vi "CRYProject Editor TS Load Open Sub.vi"(0 "Seq File Name":string, 1 "Sequence path":path) -> (7 "TS Array":T1 {"Steps"."Repeat State Array"."Start" format="%#_5g"; "Steps"."Y dB ref" format="%.1f"; "Steps"."Y data" items=["dB", "Lin"]; "Steps"."Start" format="%#_5g"}, 9 "status":bool)   [LabVIEW 2013]
uses:
  CRYSystem/Typedef Control/CRYTS.ctl
  CRYSystem/Typedef Control/CRYStep.ctl
  CRYSystem/Calibration/SubVI/CRYCal Global.vi
  CRYSystem/Misc/SubVI/CRYMisc vis settings global.vi
  CRYMainGlobal.vi
panel:
  # "Sequence Loading..."
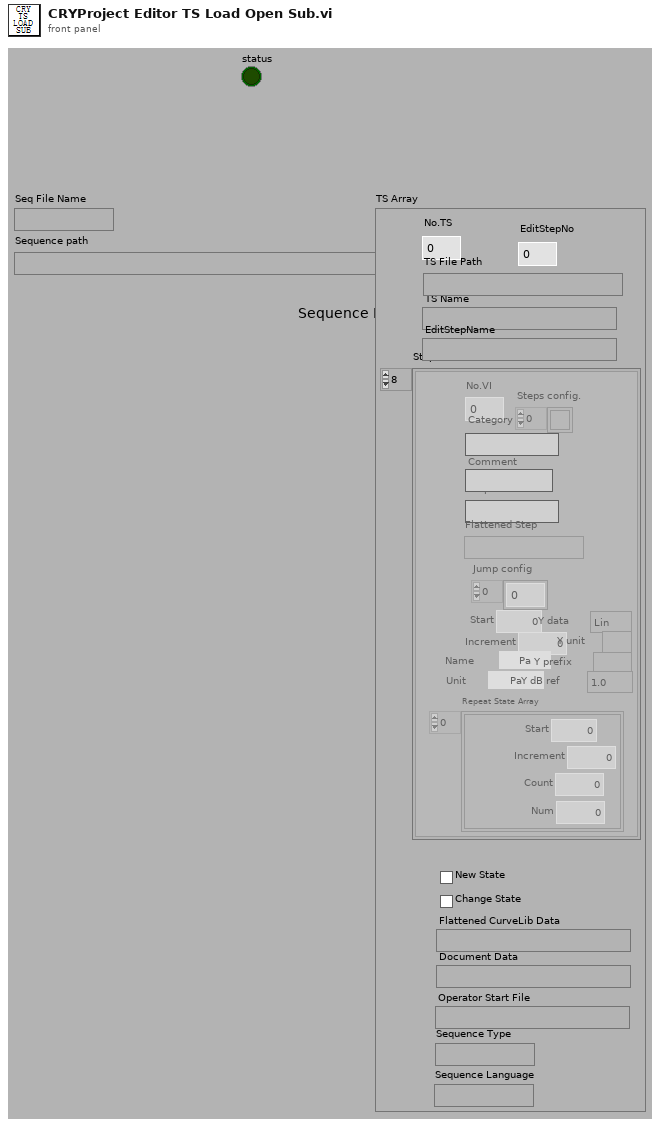
[diagram p1: front panel]
types:
  T1 = typedef "CRYTS.ctl" = cluster{"No.TS":u16, "TS File Path":path, "TS Name":string, "EditStepName":string, "Steps":T2[], "New State":bool, "Change State":bool, "Flattened CurveLib Data":string, "Document Data":string, "EditStepNo":u16, "Operator Start File":string, "Sequence Type":string, "Sequence Language":string}
  T2 = typedef "CRYStep.ctl" = cluster{"No.VI":i32, "Category":string, "StepName":string, "Seq setup flattened":string, "Comment":string, "Steps config.":bool[], "Jump config":i32[], "Start":dbl, "Increment":dbl, "Name":string, "Unit":string, "Y data":u16, "Y prefix":string, "Y dB ref":dbl, "Y unit":string, "Repeat State Array":cluster{"Start":dbl, "Increment":dbl, "Count":i32, "Num":i32}[]}
  T3 = typedef "CRYSequence Cluster.ctl" = cluster{"EditStepName":string, "Trimmed string array":string, "Flattened CurveData":string, "Document Data":string, "EditStepNo":u16, "Operator Start File":path, "Sequence Type":string, "Sequence Language":string, "Sequence Work State":string}
  T4 = cluster{"Data type":string, "Version":u16, "Dimensions":u8}
  T5 = enum16{"OK", "Yes", "YesNo", "YesNoCancel", "ReplaceAppend"}
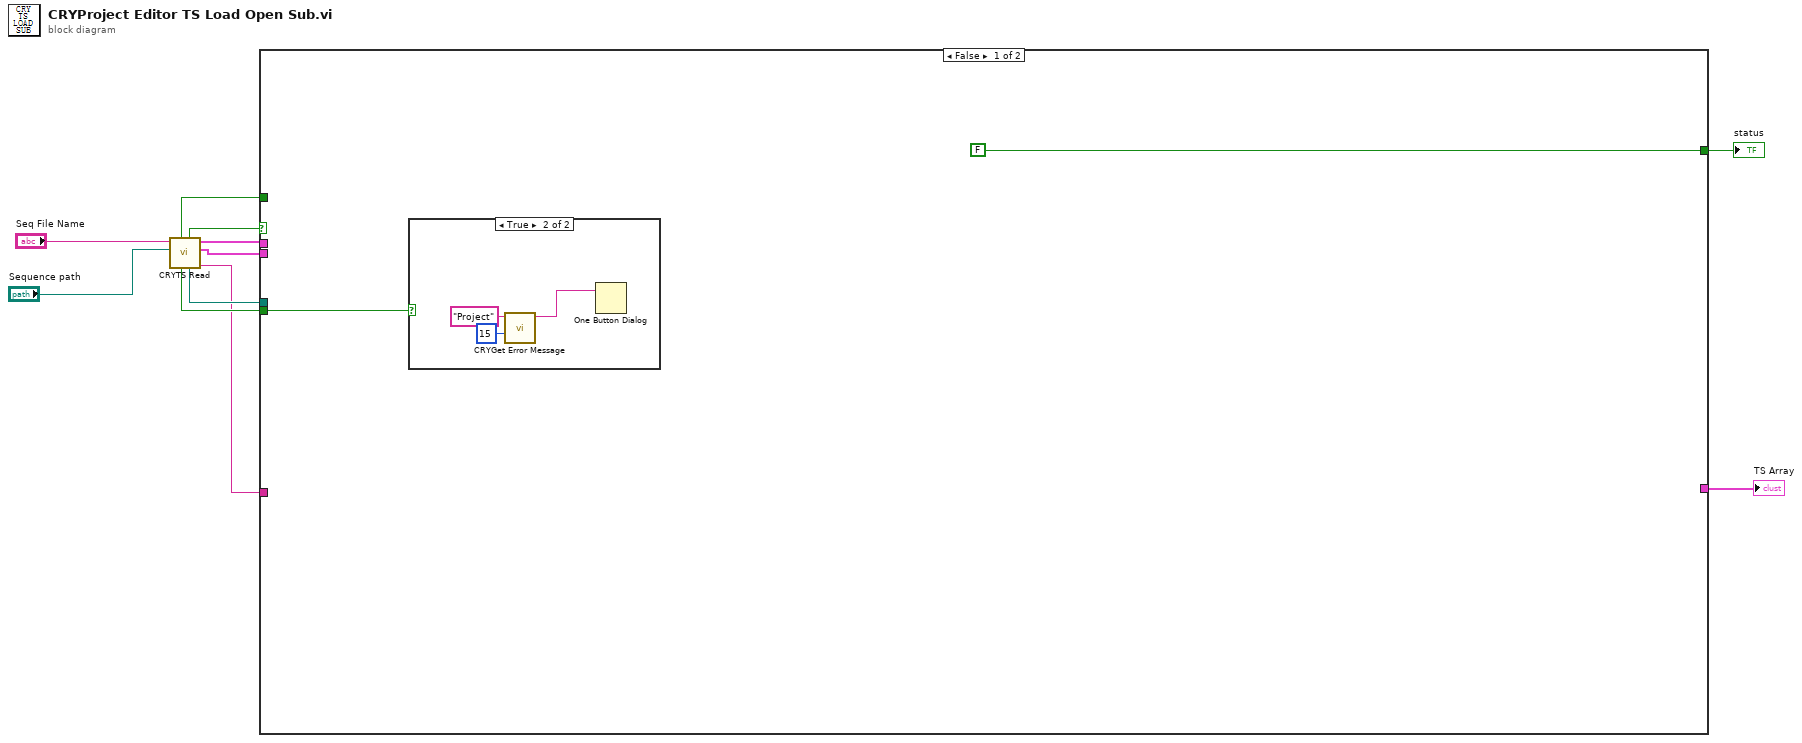
[diagram p0: block diagram]
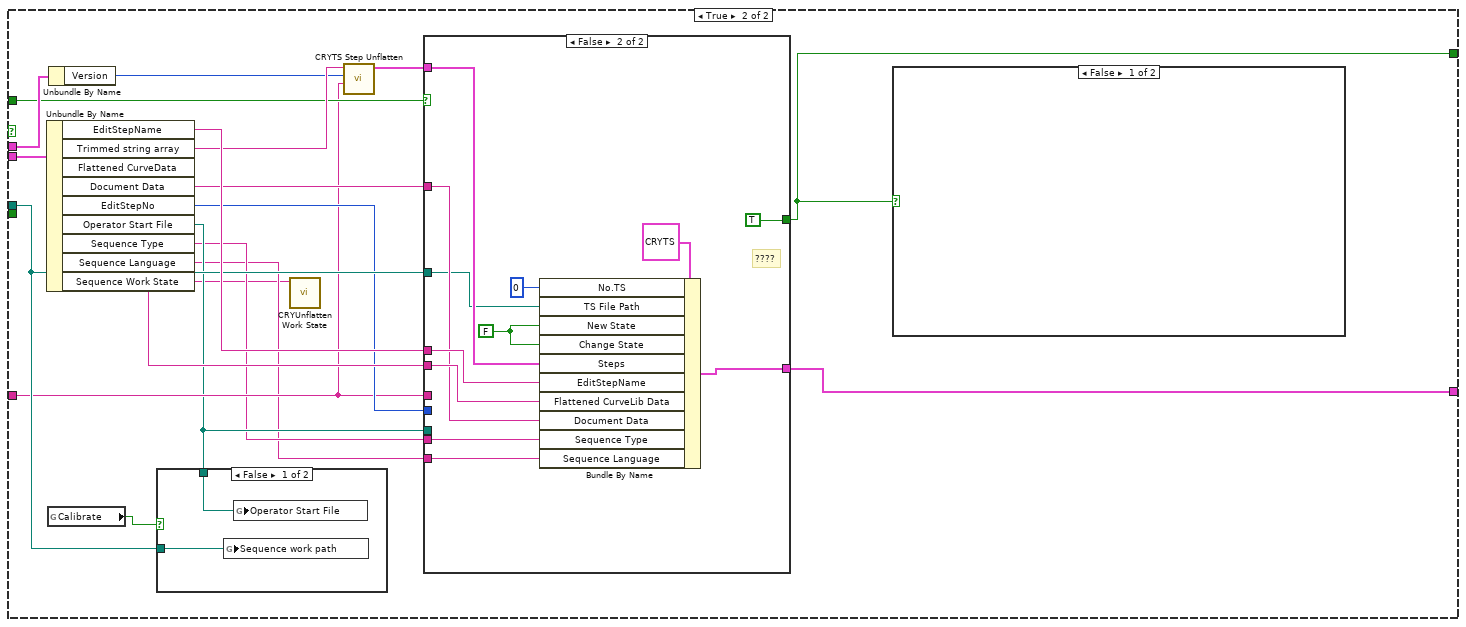
[diagram p3: hidden frame]
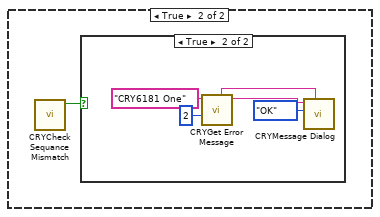
[diagram p5: hidden frame]
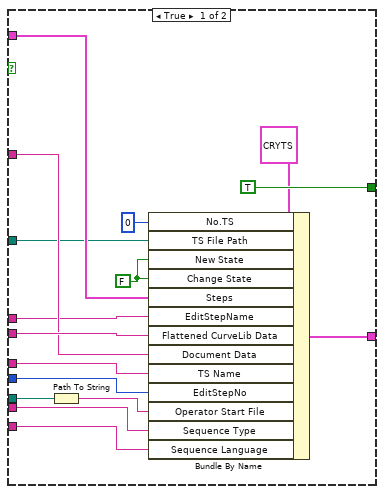
[diagram p7: hidden frame]
diagram:
  n1 = call "CRYTS Read.vi"("Sequence folder path"="Sequence path", "File Name"="Seq File Name") -> ("Sequence Name"=w4:string, "sequence list"=w6:T3, "Header info"=w8:T4, "Selected Seq Path"=w10:path, "status"=w5:bool, "Is RecentFile?"=w9:bool, "Is Replace?"=w7:bool)  [unwired: 3 out]
  n2 = case shown="False" w5 {
    tunnel: w6 -> [_ w35]
    tunnel: [FALSE ("status") w32] -> w11
    tunnel: w10 -> [_ w26]
    tunnel: w9 -> [w12 _]
    tunnel: w8 -> [_ w30]
    tunnel: w7 -> [_ w28]
    tunnel: w4 -> [_ w24]
    tunnel: [_ w17] -> w1
    frame False {
      n3 = case shown="True" w12 {
        frame False {
        }
        frame True {
          n4 = call "CRYGet Error Message.vi"("Error No"=15, "Kind"="Project") -> ("Message"=w14:string)  [unwired: 4 in, 5 out]
          n5 = One Button Dialog(message=w14) -> ()  [unwired: 2 out]
        }
      }
    }
    frame True {
      n6 = Unbundle By Name(w35) -> ("EditStepName"=w34:string, "Trimmed string array"=w31:string, "Flattened CurveData"=w33:string, "Document Data"=w27:string, "EditStepNo"=w25:u16, "Operator Start File"=w23:path, "Sequence Type"=w22:string, "Sequence Language"=w20:string, "Sequence Work State"=w19:string)
      n7 = global read "CRYCal Global.vi" "Calibrate"() -> (w18:bool)
      n8 = Unbundle By Name(w30) -> ("Version"=w29:u16)
      n9 = case shown="False" w18 {
        tunnel: w26 -> [w37 _]
        tunnel: w23 -> [w36 _]
        frame False {
          n10 = global write "CRYMainGlobal.vi" "Sequence work path"(w37) -> ()
          n11 = global write "CRYMisc vis settings global.vi" "Operator Start File"(w36) -> ()
        }
        frame True {
        }
      }
      n12 = call "CRYUnflatten Work State.vi"("Unflatten work state #"=w19) -> ()  [unwired: 9 in, 2 out]
      n13 = call "CRYTS Step Unflatten.vi"("Sequence Name"=w24, "Version"=w29, "Flattened Steps"=w31) -> ("Unflattened Steps"=w21:T2[])  [unwired: 8 out]
      n14 = case shown="False" w28 {
        tunnel: w21 -> [w59 w70]
        tunnel: [w51 w62] -> w17
        tunnel: w34 -> [w48 w68]
        tunnel: w33 -> [w58 w67]
        tunnel: [TRUE TRUE] -> w32
        tunnel: w27 -> [w53 w64]
        tunnel: w26 -> [w52 w63]
        tunnel: w24 -> [w50 _]
        tunnel: w25 -> [w49 _]
        tunnel: w23 -> [w47 _]
        tunnel: w22 -> [w45 w61]
        tunnel: w20 -> [w44 w60]
        frame True {
          w56 = FALSE ("New Sequence Flag")
          n15 = Path To String(path=w47) -> (string=w46:string)
          n16 = Bundle By Name(cluster=T1 {"No.TS"=0, "TS File Path"=path "", "TS Name"="", "EditStepName"="", "Steps"=[], "New State"=FALSE, "Change State"=FALSE, "Flattened CurveLib Data"="", "Document Data"="", "EditStepNo"=0, "Operator Start File"="", "Sequence Type"="", "Sequence Language"=""} ("Cluster"), "No.TS"=u16 0, "TS File Path"=w52, "New State"=w56, "Change State"=w56, "Steps"=w59, "EditStepName"=w48, "Flattened CurveLib Data"=w58, "Document Data"=w53, "TS Name"=w50, "EditStepNo"=w49, "Operator Start File"=w46, "Sequence Type"=w45, "Sequence Language"=w44) -> (w51:T1)
        }
        frame False {
          w71 = FALSE ("New Sequence Flag")
          # "????"
          n17 = Bundle By Name(cluster=T1 {"No.TS"=0, "TS File Path"=path "", "TS Name"="", "EditStepName"="", "Steps"=[], "New State"=FALSE, "Change State"=FALSE, "Flattened CurveLib Data"="", "Document Data"="", "EditStepNo"=0, "Operator Start File"="", "Sequence Type"="", "Sequence Language"=""} ("Cluster"), "No.TS"=u16 0, "TS File Path"=w63, "New State"=w71, "Change State"=w71, "Steps"=w70, "EditStepName"=w68, "Flattened CurveLib Data"=w67, "Document Data"=w64, "Sequence Type"=w61, "Sequence Language"=w60) -> (w62:T1)
        }
      }
      n18 = case shown="False" w32 {
        frame False {
        }
        frame True {
          n19 = call "CRYCheck Sequance Mismatch.vi"() -> ("Mismatch"=w38:bool)  [unwired: 10 in, 1 out]
          n20 = case shown="True" w38 {
            frame False {
            }
            frame True {
              n21 = call "CRYGet Error Message.vi"("Error No"=2, "Kind"="CRY6181 One") -> ("Message"=w40:string, "Window Title"=w41:string)  [unwired: 4 in, 4 out]
              n22 = call "CRYMessage Dialog.vi"("Window Title"=w41, "YesNoCancel"=T5."OK", "Message Content"=w40) -> ()  [unwired: 7 in, 2 out]
            }
          }
        }
      }
    }
  }
  "status" <- w11
  "TS Array" <- w1
